vi "Set Camera Zoom Level.vi"(8 "error in (no error)":errorcluster, 11 "Zoom Level":T1=enum."Close") -> (0 "error out":errorcluster)   [LabVIEW 2026]
uses:
  Camera/Zoom Level.ctl
  Re-use Libraries/Minimal Actor Framework/Messaging/Message/Message.lvclass/Message.ctl
  Globals.vi
  Re-use Libraries/Minimal Actor Framework/Messaging/Message/Message.lvclass
  Main Controller Actor API.lvclass
  Camera/Camera.lvclass
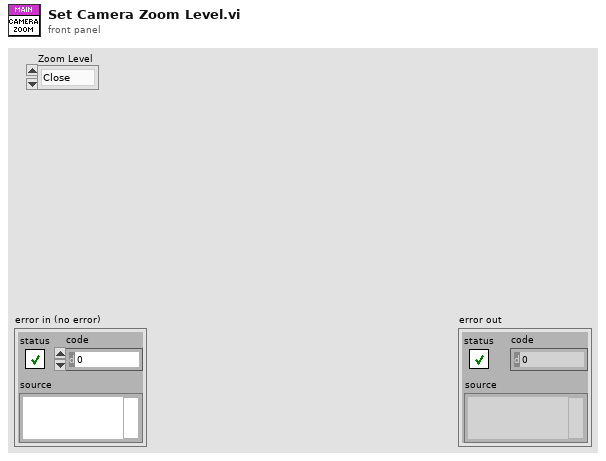
[diagram p1: front panel]
types:
  T1 = typedef "Camera.lvclass/Zoom Level.ctl" = enum16{"Far", "Medium", "Close"}
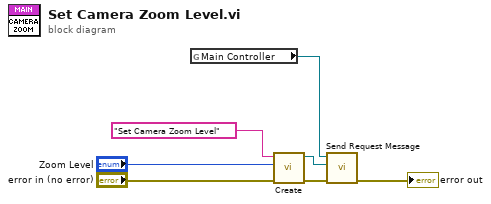
[diagram p0: block diagram]
diagram:
  n1 = global read "Globals.vi" "Main Controller"() -> (w4:refnum<class "Main Controller Actor API.lvclass">)
  n2 = call "Create.vi"("error in (no error)"="error in (no error)", "Data"="Zoom Level", "Name"="Set Camera Zoom Level" ("Parameter")) -> ("error out"=w5:errorcluster, "Message out"=w6:refnum<class "Message.lvclass">)  [unwired: 7 in]
  n3 = call-dynamic "Send Request Message.vi"("error in (no error)"=w5, "Message"=w6, "Actor API in"=w4) -> ("error out"=→"error out":errorcluster)  [unwired: 8 in]
